vi "ssh_test.vi"(8 "error in":errorcluster, 10 "SSH Disabled?":bool=TRUE, 11 "VISA resource name":refnum<visa-resource-name>="COM56") -> (0 "error out":errorcluster, 1 "Script output":string, 2 "Firewall settings ok?":bool, 3 "DHCP Setting OK?":bool)   [LabVIEW 2013]
panel:
  out "pscp timed out?":bool
  out "standard error pscp":string
  out "standard output pscp":string
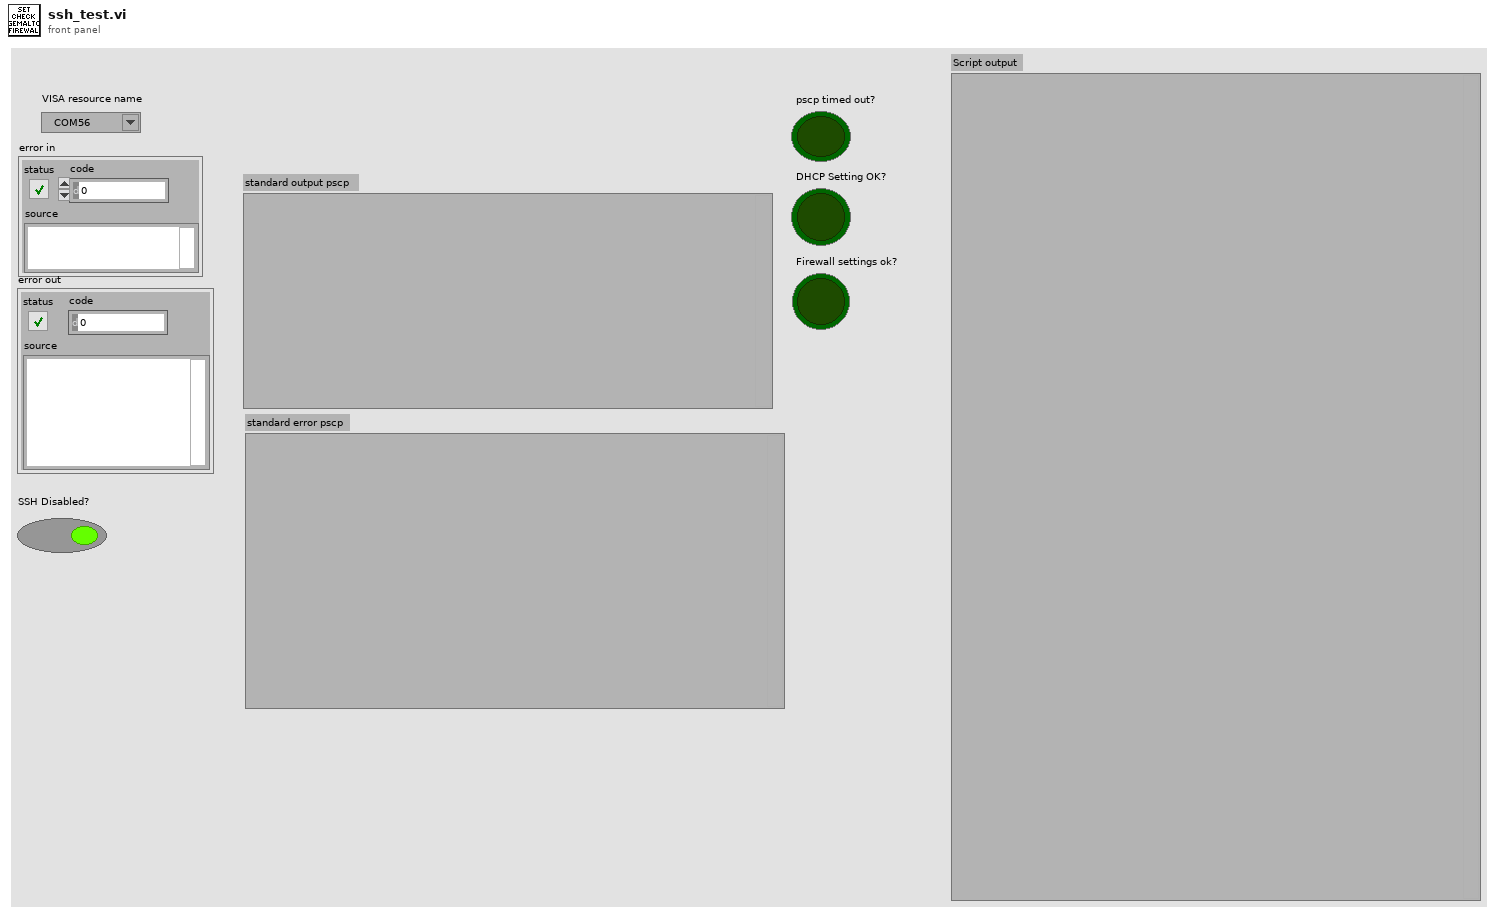
[diagram p1: front panel]
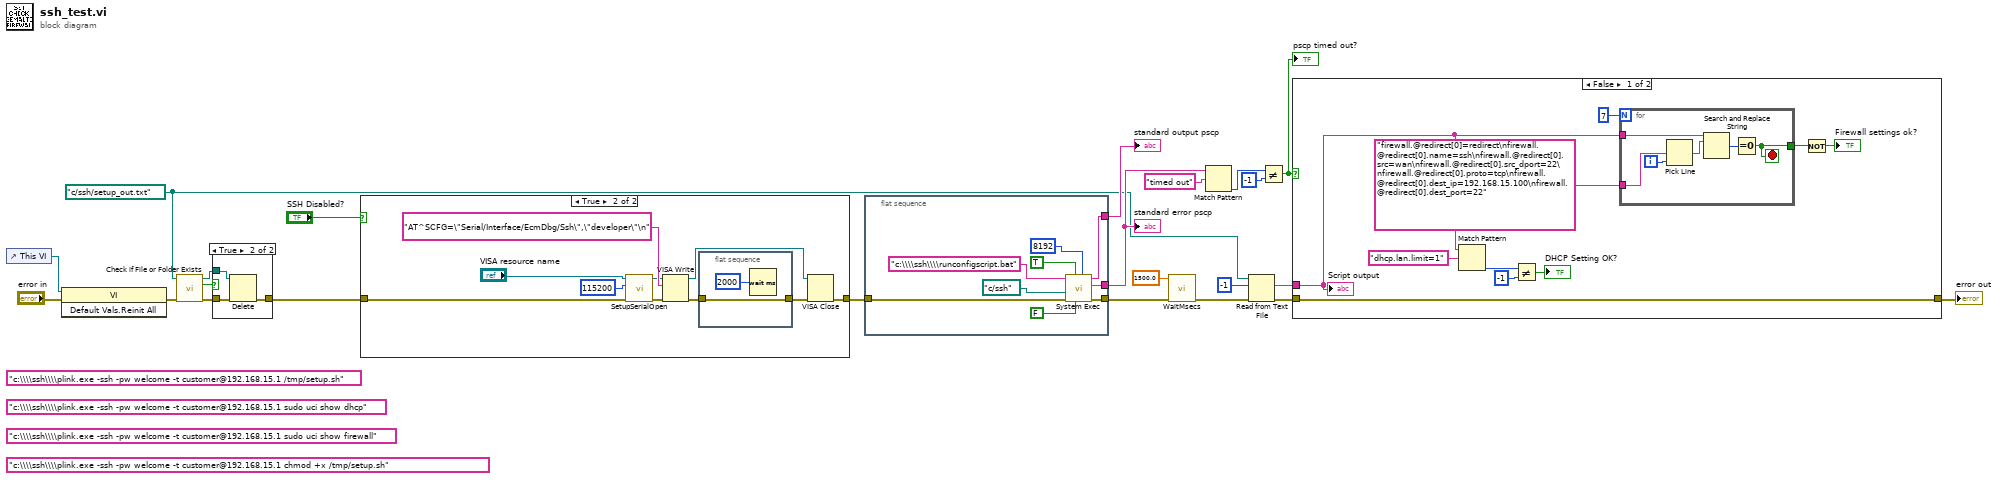
[diagram p0: block diagram]
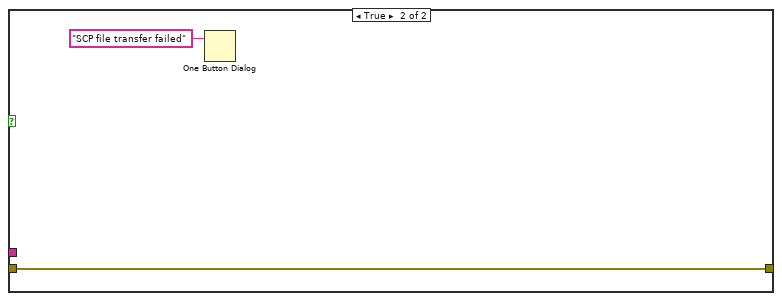
[diagram p3: hidden frame]
diagram:
  w8 = path "c:/ssh/setup_out.txt" ("file (use dialog)")
  (unwired) "c:\\\\ssh\\\\plink.exe -ssh -pw welcome -t customer@192.168.15.1 sudo uci show firewall" ("string")
  (unwired) "c:\\\\ssh\\\\plink.exe -ssh -pw welcome -t customer@192.168.15.1 sudo uci show dhcp" ("string")
  (unwired) "c:\\\\ssh\\\\plink.exe -ssh -pw welcome -t customer@192.168.15.1 /tmp/setup.sh" ("string")
  (unwired) "c:\\\\ssh\\\\plink.exe -ssh -pw welcome -t customer@192.168.15.1 chmod +x /tmp/setup.sh"
  n1 = control-ref of="This VI"() -> (w19:refnum<vi>)
  n2 = invoke class="VI" method="Default Vals.Reinit All"(reference=w19, error in="error in") -> (error out=w7:errorcluster)  [unwired: 1 in, 2 out]
  n3 = call <vilib>:"Check if File or Folder Exists.vi"("error in (no error)"=w7, "path"=w8) -> ("error out"=w5:errorcluster, "file or folder exists?"=w6:bool, "dup path"=w4:path)  [unwired: 7 in]
  n4 = case shown="True" w6 {
    tunnel: [w24 w27] -> w9
    tunnel: w5 -> [w24 w26]
    tunnel: w4 -> [_ w25]
    frame False {
    }
    frame True {
      n5 = Delete(path (use dialog)=w25, error in=w26) -> (error out=w27:errorcluster)  [unwired: 3 in, 2 out]
    }
  }
  n6 = case shown="True" "SSH Disabled?" {
    tunnel: w9 -> [w28 w32]
    tunnel: [w28 w36] -> w22
    frame False {
    }
    frame True {
      n7 = call "SetupSerialOpen.vi"("error in (no error)"=w32, "Baud"=u32 115200 ("baud rate (9600)"), "VISA Refnum in"="VISA resource name") -> ("error out"=w30:errorcluster, "VISA session"=w29:refnum<visa-resource-name>)  [unwired: 7 in]
      n8 = VISA Write(VISA resource name=w29, write buffer="AT^SCFG=\"Serial/Interface/EcmDbg/Ssh\",\"developer\"\n", error in (no error)=w30) -> (VISA resource name out=w37:refnum<visa-resource-name>, error out=w34:errorcluster)  [unwired: 1 out]
      n9 = flat-sequence {
        tunnel: [w39] -> w35
        tunnel: w34 -> [w39]
        frame #0 {
          n10 = Wait (ms)(milliseconds to wait=u32 2000) -> ()  [unwired: 1 out]
        }
      }
      n11 = VISA Close(VISA resource name=w37, error in (no error)=w35) -> (error out=w36:errorcluster)
    }
  }
  n12 = flat-sequence {
    tunnel: [w49] -> w23
    tunnel: w22 -> [w48]
    tunnel: [w45] -> w17
    tunnel: [w44] -> w3
    frame #0 {
      n13 = call <vilib>:"System Exec.vi"("expected output size  (4096)"=u32 8192, "run minimized? (F)"=FALSE, "wait until completion? (T)"=TRUE, "error in (no error)"=w48, "working directory"=path "c:/ssh", "command line"="c:\\\\ssh\\\\runconfigscript.bat") -> ("error out"=w44:errorcluster, "standard error"=w45:string, "standard output"=w49:string)  [unwired: 2 in, 1 out]
    }
  }
  n14 = call "WaitMsecs.vi"("error in (no error)"=w3, "Wait Msecs"=1500.0) -> ("error out"=w2:errorcluster)  [unwired: 9 in]
  n15 = Match Pattern(string=w17, regular expression="timed out") -> (offset past match=w15:i32)  [unwired: 1 in, 3 out]
  n16 = Read from Text File(file (use dialog)=w8, count=-1, error in=w2) -> (text=w10:string, error out=w11:errorcluster)  [unwired: 1 in, 2 out]
  n17 = Not Equal?(x=w15, y=-1) -> (x != y?=w13:bool)
  "pscp timed out?" <- w13
  n18 = case shown="False" w13 {
    tunnel: w11 -> [w51 w67]
    tunnel: [w51 w67] -> w21
    tunnel: w10 -> [w50 _]
    frame False {
      n19 = Match Pattern(string=w50, regular expression="dhcp.lan.limit=1") -> (offset past match=w53:i32)  [unwired: 1 in, 3 out]
      n20 = Not Equal?(x=w53, y=-1) -> (x != y?=→"DHCP Setting OK?":bool)
      n21 = for {
        N: 7 -> [_]
        tunnel: "firewall.@redirect[0]=redirect\nfirewall.@redirect[0].name=ssh\nfirewall.@redirect[0].src=wan\nfirewall.@redirect[0].src_dport=22\nfirewall.@redirect[0].proto=tcp\nfirewall.@redirect[0].dest_ip=192.168.15.100\nfirewall.@redirect[0].dest_port=22" -> [w65]
        tunnel: [w61] -> w57
        tunnel: w50 -> [w60]
        i -> [w64]
        stop <- w61 stop-if-true
        n22 = Pick Line(multi-line string=w65, line index=w64) -> (output string=w63:string)  [unwired: 1 in]
        n23 = Search and Replace String(input string=w60, search string=w63) -> (number of replacements=w62:i32)  [unwired: 6 in, 3 out]
        n24 = Equal To 0?(x=w62) -> (x = 0?=w61:bool)
      }
      n25 = Not(x=w57) -> (.not. x?=→"Firewall settings ok?":bool)
      "Script output" <- w50
    }
    frame True {
      n26 = One Button Dialog(message="SCP file transfer failed") -> ()  [unwired: 1 in, 1 out]
    }
  }
  "error out" <- w21
  "standard output pscp" <- w23
  "standard error pscp" <- w17
